vi "KE6221 -- Set Square Or Ramp Wave Params.vi"(0 "Resource In":refnum<visa-resource-name>, 1 "Check For SCPI Errors? (T)":bool=TRUE, 5 "Wave Type In":T2, 7 "Square Or Ramp Wave Params In":T3={"Frequency (Hz)"=1000.0, "Amplitude (A)"=0.001, "Offset (A)"=0.0, "Duty Cycle (%)"=50.0, "Ranging Mode"=enum."Best", "Fixed Range"=enum."2mA", "Playback Mode"=enum."Time", "Time (s)"=1.0, "Num Cycles"=1.0, "Phase\nMarker?"=FALSE, "Phase Marker (deg)"=180.0, "Trig Link Line"=enum."1"} {"Duty Cycle (%)" min=0.0 max=100.0 format="%.3p"; "Offset (A)" min=-0.105 max=0.105 format="%.4p"; "Num Cycles" min=0.001 max=99999999900.0 format="%.3p"; "Time (s)" min=1e-07 max=999999.999 format="%.3p"; "Phase Marker (deg)" min=0.0 max=360.0 format="%.3f"; "Amplitude (A)" min=2e-12 max=0.105 format="%.3p"; "Frequency (Hz)" min=0.001 max=100000.0 format="%.3p"}, 11 "error in (no error)":errorcluster, 12 "Read Back Set Values? (T)":bool=TRUE) -> (4 "Resource Out (dupl)":refnum<visa-resource-name>, 8 "Square Or Ramp Wave Params Out":T3={"Frequency (Hz)"=1000.0, "Amplitude (A)"=0.001, "Offset (A)"=0.0, "Duty Cycle (%)"=50.0, "Ranging Mode"=enum."Best", "Fixed Range"=enum."2mA", "Playback Mode"=enum."Time", "Time (s)"=1.0, "Num Cycles"=1.0, "Phase\nMarker?"=FALSE, "Phase Marker (deg)"=180.0, "Trig Link Line"=enum."1"} {"Duty Cycle (%)" min=0.0 max=100.0 format="%.3p"; "Offset (A)" min=-0.105 max=0.105 format="%.4p"; "Num Cycles" min=0.001 max=99999999900.0 format="%.3p"; "Time (s)" min=1e-07 max=999999.999 format="%.3p"; "Phase Marker (deg)" min=0.0 max=360.0 format="%.3f"; "Amplitude (A)" min=2e-12 max=0.105 format="%.3p"; "Frequency (Hz)" min=0.001 max=100000.0 format="%.3p"}, 15 "error out":errorcluster)   [LabVIEW 2019, in "Keithley 622x.lvlib"]
doc: "Sets the parameters for either a square wave or a ramp wave. The user must specify which type of waveform he wants (Square or Ramp). Note that this VI can only be used with the 6221, since the 6220 doesn't support this feature."
uses:
  Keithley 622x.lvlib
  Typedefs/KE6221 -- Wave Square Or Ramp Wave Params.ctl
  Low Level/Typedefs/KE6221 -- Wave Frequency.ctl
  Low Level/Typedefs/KE6221 -- Wave Amplitude.ctl
  Source/Typedefs/KE622x -- Current Level.ctl
  Low Level/Typedefs/KE6221 -- Wave Duty Cycle.ctl
  Low Level/Typedefs/KE6221 -- Wave Ranging Mode.ctl
  Source/Typedefs/KE622x -- Current Ranges.ctl
  Low Level/Typedefs/KE6221 -- Wave Playback Mode.ctl
  Low Level/Typedefs/KE6221 -- Wave Playback Time.ctl
  Low Level/Typedefs/KE6221 -- Wave Playback Num Cycles.ctl
  Low Level/Typedefs/KE6221 -- Wave Phase Marker.ctl
  Trigger/Low Level/Typedefs/KE622x -- Trig Link Line.ctl
  Typedefs/KE6221 -- Wave Square Or Ramp Wave Select.ctl
  Low Level/Typedefs/KE6221 -- Wave Type.ctl
  Source/Typedefs/KE622x -- Current Range.ctl
panel:
  out "Wave Type Out":T1=enum."Square"
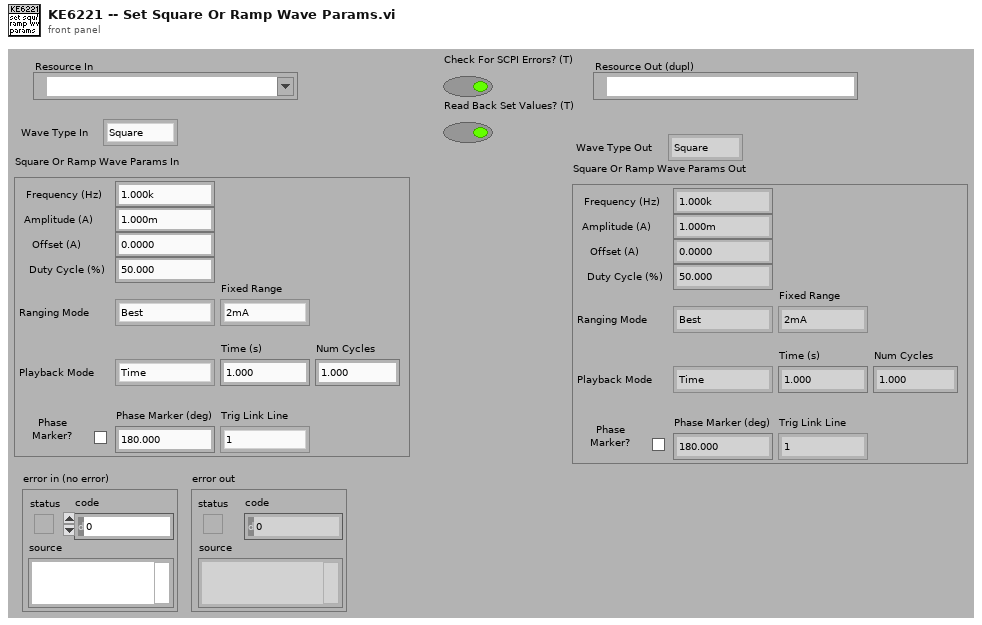
[diagram p1: front panel]
types:
  T1 = typedef "Keithley 622x.lvlib/KE6221 -- Wave Type.ctl" = enum16{"Sinusoid", "Square", "Ramp", "Arbitrary 0", "Arbitrary 1", "Arbitrary 2", "Arbitrary 3", "Arbitrary 4"}
  T2 = typedef "Keithley 622x.lvlib/KE6221 -- Wave Square Or Ramp Wave Select.ctl" = enum16{"Square", "Ramp"}
  T3 = typedef "Keithley 622x.lvlib/KE6221 -- Wave Square Or Ramp Wave Params.ctl" = cluster{"Frequency (Hz)":T4, "Amplitude (A)":T5, "Offset (A)":T6, "Duty Cycle (%)":T7, "Ranging Mode":T8, "Fixed Range":T9, "Playback Mode":T10, "Time (s)":T11, "Num Cycles":T12, "Phase\nMarker?":bool, "Phase Marker (deg)":T13, "Trig Link Line":T14}
  T4 = typedef "Keithley 622x.lvlib/KE6221 -- Wave Frequency.ctl" = dbl
  T5 = typedef "Keithley 622x.lvlib/KE6221 -- Wave Amplitude.ctl" = dbl
  T6 = typedef "Keithley 622x.lvlib/KE622x -- Current Level.ctl" = dbl
  T7 = typedef "Keithley 622x.lvlib/KE6221 -- Wave Duty Cycle.ctl" = dbl
  T8 = typedef "Keithley 622x.lvlib/KE6221 -- Wave Ranging Mode.ctl" = enum16{"Best", "Fixed"}
  T9 = typedef "Keithley 622x.lvlib/KE622x -- Current Ranges.ctl" = enum16{"2nA", "20nA", "200nA", "2uA", "20uA", "200uA", "2mA", "20mA", "100mA"}
  T10 = typedef "Keithley 622x.lvlib/KE6221 -- Wave Playback Mode.ctl" = enum16{"Time", "Num Cycles"}
  T11 = typedef "Keithley 622x.lvlib/KE6221 -- Wave Playback Time.ctl" = dbl
  T12 = typedef "Keithley 622x.lvlib/KE6221 -- Wave Playback Num Cycles.ctl" = dbl
  T13 = typedef "Keithley 622x.lvlib/KE6221 -- Wave Phase Marker.ctl" = dbl
  T14 = typedef "Keithley 622x.lvlib/KE622x -- Trig Link Line.ctl" = enum16{"1", "2", "3", "4", "5", "6"}
  T15 = typedef "Keithley 622x.lvlib/KE622x -- Current Range.ctl" = cluster{"Auto Range?":bool, "Man / Selected\nRange":T9}
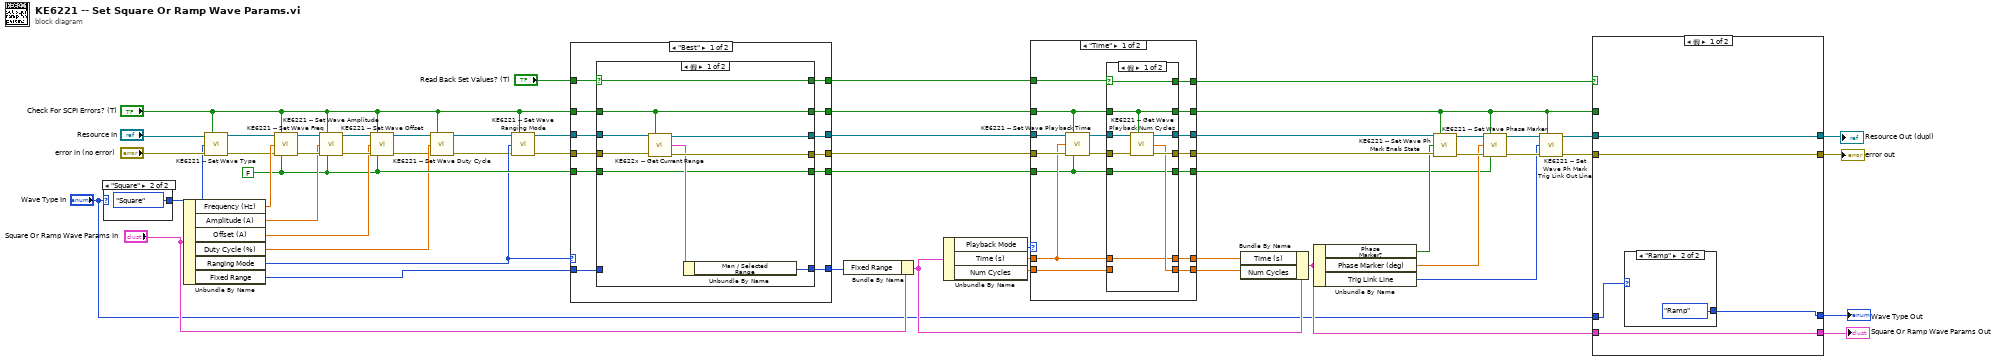
[diagram p0: block diagram]
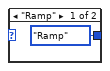
[diagram p2: hidden frame]
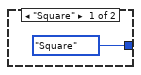
[diagram p3: hidden frame]
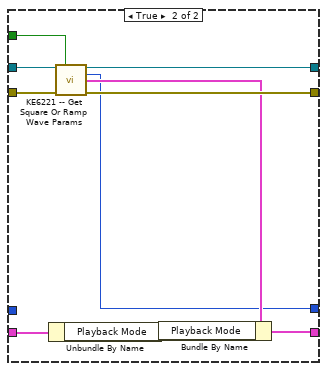
[diagram p4: hidden frame]
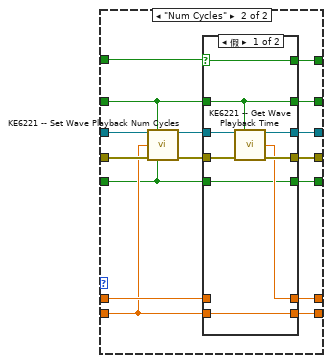
[diagram p6: hidden frame]
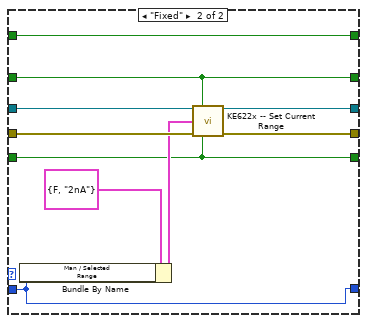
[diagram p9: hidden frame]
diagram:
  w26 = FALSE
  n1 = case shown="\"Square\"" "Wave Type In" {
    tunnel: [KE6221_--_Wave_Type."Ramp" ("Wave Type") KE6221_--_Wave_Type."Square" ("Wave Type")] -> w5
    frame "Ramp" {
    }
    frame "Square" {
    }
  }
  n2 = Unbundle By Name("Square Or Ramp Wave Params In") -> ("Frequency (Hz)"=w47:T4, "Amplitude (A)"=w46:T5, "Offset (A)"=w45:T6, "Duty Cycle (%)"=w15:T7, "Ranging Mode"=w16:T8, "Fixed Range"=w44:T9)
  n3 = call "KE6221 -- Set Wave Type.vi"("Resource In"="Resource In", "Check For SCPI Errors? (T)"="Check For SCPI Errors? (T)", "Wave Type"=w5, "error in (no error)"="error in (no error)") -> ("Resource Out (dupl)"=w7:refnum<visa-resource-name>, "error out"=w8:errorcluster)  [unwired: 10 in]
  n4 = call "KE6221 -- Set Wave Freq.vi"("Resource In"=w7, "Check For SCPI Errors? (T)"="Check For SCPI Errors? (T)", "Wave Frequency In (Hz)"=w47, "error in (no error)"=w8, "Read Back Set Value? (T)"=w26) -> ("Resource Out (dupl)"=w57:refnum<visa-resource-name>, "error out"=w56:errorcluster)  [unwired: 8 in, 1 out]
  n5 = call "KE6221 -- Set Wave Amplitude.vi"("Resource In"=w57, "Check For SCPI Errors? (T)"="Check For SCPI Errors? (T)", "Wave Amplitude In"=w46, "error in (no error)"=w56, "Read Back Set Value? (T)"=w26) -> ("Resource Out (dupl)"=w53:refnum<visa-resource-name>, "error out"=w52:errorcluster)  [unwired: 8 in, 1 out]
  n6 = call "KE6221 -- Set Wave Offset.vi"("Resource In"=w53, "Check For SCPI Errors? (T)"="Check For SCPI Errors? (T)", "Wave Offset In (A)"=w45, "error in (no error)"=w52, "Read Back Set Value? (T)"=w26) -> ("Resource Out (dupl)"=w17:refnum<visa-resource-name>, "error out"=w14:errorcluster)  [unwired: 8 in, 1 out]
  n7 = call "KE6221 -- Set Wave Duty Cycle.vi"("Resource In"=w17, "Check For SCPI Errors? (T)"="Check For SCPI Errors? (T)", "Duty Cycle In (%)"=w15, "error in (no error)"=w14) -> ("Resource Out (dupl)"=w13:refnum<visa-resource-name>, "error out"=w12:errorcluster)  [unwired: 9 in, 1 out]
  n8 = call "KE6221 -- Set Wave Ranging Mode.vi"("Resource In"=w13, "Check For SCPI Errors? (T)"="Check For SCPI Errors? (T)", "Ranging Mode"=w16, "error in (no error)"=w12) -> ("Resource Out (dupl)"=w55:refnum<visa-resource-name>, "error out"=w54:errorcluster)  [unwired: 10 in]
  n9 = case shown="\"Best\"" w16 {
    tunnel: w55 -> [w70 w96]
    tunnel: w54 -> [w69 w95]
    tunnel: [w66 w94] -> w41
    tunnel: [w67 w93] -> w38
    tunnel: "Check For SCPI Errors? (T)" -> [w68 w89]
    tunnel: w44 -> [w63 w88]
    tunnel: "Read Back Set Values? (T)" -> [w71 w90]
    tunnel: [w65 w89] -> w37
    tunnel: [w64 w90] -> w36
    tunnel: [w62 w88] -> w35
    tunnel: w26 -> [w61 w87]
    tunnel: [w60 w87] -> w25
    frame "Best" {
      n10 = case shown="假" w71 {
        selector: w71 -> [w75 w86]
        tunnel: w70 -> [w80 w84]
        tunnel: w69 -> [w79 w83]
        tunnel: w68 -> [w76 w85]
        tunnel: [w78 w83] -> w67
        tunnel: [w77 w84] -> w66
        tunnel: [w76 w85] -> w65
        tunnel: [w75 w86] -> w64
        tunnel: w63 -> [_ w82]
        tunnel: [w73 w82] -> w62
        tunnel: w61 -> [w72 w81]
        tunnel: [w72 w81] -> w60
        frame False {
          n11 = call "KE622x -- Get Current Range.vi"("Resource In"=w80, "Check For SCPI Errors? (T)"=w76, "error in (no error)"=w79) -> ("Resource Out (dupl)"=w77:refnum<visa-resource-name>, "Current Range"=w74:T15, "error out"=w78:errorcluster)  [unwired: 10 in]
          n12 = Unbundle By Name(w74) -> ("Man / Selected\nRange"=w73:T9)
        }
        frame True {
        }
      }
    }
    frame "Fixed" {
      n13 = Bundle By Name(cluster=T15 {"Auto Range?"=FALSE, "Man / Selected\nRange"=enum."2nA"} ("Current Range In"), "Man / Selected\nRange"=w88) -> (w91:T15)
      n14 = call "KE622x -- Set Current Range.vi"("Resource In"=w96, "Check For SCPI Errors? (T)"=w89, "Current Range In"=w91, "error in (no error)"=w95, "Read Back Set Values? (T)"=w87) -> ("Resource Out (dupl)"=w94:refnum<visa-resource-name>, "error out"=w93:errorcluster)  [unwired: 8 in, 1 out]
    }
  }
  n15 = Bundle By Name(cluster="Square Or Ramp Wave Params In", "Fixed Range"=w35) -> (w34:T3)
  n16 = Unbundle By Name(w34) -> ("Playback Mode"=w42:T10, "Time (s)"=w40:T11, "Num Cycles"=w39:T12)
  n17 = case shown="\"Time\"" w42 {
    tunnel: w41 -> [w112 w144]
    tunnel: w40 -> [w101 w135]
    tunnel: w39 -> [w103 w133]
    tunnel: w38 -> [w111 w143]
    tunnel: w37 -> [w107 w139]
    tunnel: w36 -> [w110 w142]
    tunnel: [w102 w132] -> w32
    tunnel: [w106 w138] -> w20
    tunnel: [w105 w137] -> w31
    tunnel: [w104 w136] -> w30
    tunnel: [w100 w134] -> w33
    tunnel: w25 -> [w99 w131]
    tunnel: [w98 w130] -> w24
    tunnel: [w97 w129] -> w23
    frame "Time" {
      n18 = call "KE6221 -- Set Wave Playback Time.vi"("Resource In"=w112, "Check For SCPI Errors? (T)"=w107, "Playback Time (s) In"=w101, "error in (no error)"=w111, "Read Back Set Value? (T)"=w99) -> ("Resource Out (dupl)"=w109:refnum<visa-resource-name>, "error out"=w108:errorcluster)  [unwired: 8 in, 1 out]
      n19 = case shown="假" w110 {
        selector: w110 -> [w113 w122]
        tunnel: w109 -> [w121 w126]
        tunnel: w108 -> [w120 w127]
        tunnel: w107 -> [w119 w128]
        tunnel: [w119 w128] -> w106
        tunnel: [w118 w127] -> w104
        tunnel: [w117 w126] -> w105
        tunnel: w103 -> [_ w125]
        tunnel: [w116 w125] -> w102
        tunnel: w101 -> [w115 w124]
        tunnel: [w115 w124] -> w100
        tunnel: w99 -> [w114 w123]
        tunnel: [w114 w123] -> w98
        tunnel: [w113 w122] -> w97
        frame False {
          n20 = call "KE6221 -- Get Wave Playback Num Cycles.vi"("Resource In"=w121, "Check For SCPI Errors? (T)"=w119, "error in (no error)"=w120) -> ("Resource Out (dupl)"=w117:refnum<visa-resource-name>, "Num Cycles"=w116:T12, "error out"=w118:errorcluster)  [unwired: 10 in]
        }
        frame True {
        }
      }
    }
    frame "Num Cycles" {
      n21 = call "KE6221 -- Set Wave Playback Num Cycles.vi"("Resource In"=w144, "Check For SCPI Errors? (T)"=w139, "Num Cycles In"=w133, "error in (no error)"=w143, "Read Back Set Value? (T)"=w131) -> ("Resource Out (dupl)"=w141:refnum<visa-resource-name>, "error out"=w140:errorcluster)  [unwired: 8 in, 1 out]
      n22 = case shown="假" w142 {
        selector: w142 -> [w145 w154]
        tunnel: w141 -> [w153 w158]
        tunnel: w140 -> [w152 w159]
        tunnel: w139 -> [w151 w160]
        tunnel: [w151 w160] -> w138
        tunnel: [w150 w159] -> w136
        tunnel: [w149 w158] -> w137
        tunnel: w135 -> [_ w157]
        tunnel: [w148 w157] -> w134
        tunnel: w133 -> [w147 w156]
        tunnel: [w147 w156] -> w132
        tunnel: w131 -> [w146 w155]
        tunnel: [w146 w155] -> w130
        tunnel: [w145 w154] -> w129
        frame False {
          n23 = call "KE6221 -- Get Wave Playback Time.vi"("Resource In"=w153, "Check For SCPI Errors? (T)"=w151, "error in (no error)"=w152) -> ("Resource Out (dupl)"=w149:refnum<visa-resource-name>, "Playback Time (s)"=w148:T11, "error out"=w150:errorcluster)  [unwired: 10 in]
        }
        frame True {
        }
      }
    }
  }
  n24 = Bundle By Name(cluster=w34, "Time (s)"=w33, "Num Cycles"=w32) -> (w19:T3)
  n25 = Unbundle By Name(w19) -> ("Phase\nMarker?"=w29:bool, "Phase Marker (deg)"=w28:T13, "Trig Link Line"=w27:T14)
  n26 = call "KE6221 -- Set Wave Ph Mark Enab State.vi"("Resource In"=w31, "Check For SCPI Errors? (T)"=w20, "Phase Marker Enabled?"=w29, "error in (no error)"=w30) -> ("Resource Out (dupl)"=w51:refnum<visa-resource-name>, "error out"=w50:errorcluster)  [unwired: 10 in]
  n27 = call "KE6221 -- Set Wave Phase Marker.vi"("Resource In"=w51, "Check For SCPI Errors? (T)"=w20, "Phase Marker In (deg)"=w28, "error in (no error)"=w50, "Read Back Set Value? (T)"=w24) -> ("Resource Out (dupl)"=w49:refnum<visa-resource-name>, "error out"=w48:errorcluster)  [unwired: 8 in, 1 out]
  n28 = call "KE6221 -- Set Wave Ph Mark Trig Link Out Line.vi"("Resource In"=w49, "Check For SCPI Errors? (T)"=w20, "Trig Link Out Line"=w27, "error in (no error)"=w48) -> ("Resource Out (dupl)"=w22:refnum<visa-resource-name>, "error out"=w21:errorcluster)  [unwired: 10 in]
  n29 = case shown="假" w23 {
    tunnel: w22 -> [w164 w177]
    tunnel: w21 -> [w163 w176]
    tunnel: w20 -> [_ w175]
    tunnel: [w164 w174] -> w4
    tunnel: [w163 w173] -> w3
    tunnel: w19 -> [w165 w172]
    tunnel: [w165 w169] -> w11
    tunnel: [w161 w168] -> w2
    tunnel: "Wave Type In" -> [w162 _]
    frame False {
      n30 = case shown="\"Ramp\"" w162 {
        tunnel: [KE6221_--_Wave_Type."Square" ("Wave Type") KE6221_--_Wave_Type."Ramp" ("Wave Type")] -> w161
        frame "Square" {
        }
        frame "Ramp" {
        }
      }
    }
    frame True {
      n31 = Unbundle By Name(w172) -> ("Playback Mode"=w170:T10)
      n32 = call "KE6221 -- Get Square Or Ramp Wave Params.vi"("Resource In"=w177, "Check For SCPI Errors? (T)"=w175, "error in (no error)"=w176) -> ("Resource Out (dupl)"=w174:refnum<visa-resource-name>, "Wave Type"=w168:T1, "Square Or Ramp Wave Params"=w171:T3, "error out"=w173:errorcluster)  [unwired: 9 in]
      n33 = Bundle By Name(cluster=w171, "Playback Mode"=w170) -> (w169:T3)
    }
  }
  "Resource Out (dupl)" <- w4
  "error out" <- w3
  "Square Or Ramp Wave Params Out" <- w11
  "Wave Type Out" <- w2
